vi "LJUD_ListAll.vi"(8 "error in":errorcluster, 9 "ConnectionType":i32=1, 10 "DeviceType":i32=9) -> (0 "error out":errorcluster, 1 "SerialNumbers":i32[](array[numeric]), 2 "NumFound":i32=2, 5 "Addresses":i32[](array[numeric]), 7 "IDs":i32[](array[numeric]))   [LabVIEW 2021]
doc: "Returns all the devices found of a given DeviceType and\nConnectionType. \n\nDocumented in Section 4.2 of the device's datasheet.\n\nDeviceType: LJ_dtU3=3, LJ_dtU6=6, LJ_dtUE9=9\n\nConnectionType: LJ_ctUSB=1, LJ_ctETHERNET=2"
uses:
  labjackud.dll
panel:
  # "Returns all the devices found of a given DeviceType and\nConnectionType. \n\nDocumented in Section 4.2 of the device's datasheet.\n\nDeviceType:  LJ_dtU3=3, LJ_dtU6=6, LJ_dtUE9=9\n\nConnectionType:  LJ_ctUSB=1, LJ_ctETHERNET=2"
  # "U3 = 3\nU6 = 6\nUE9 = 9\n \nUSB = 1\nETHERNET = 2"
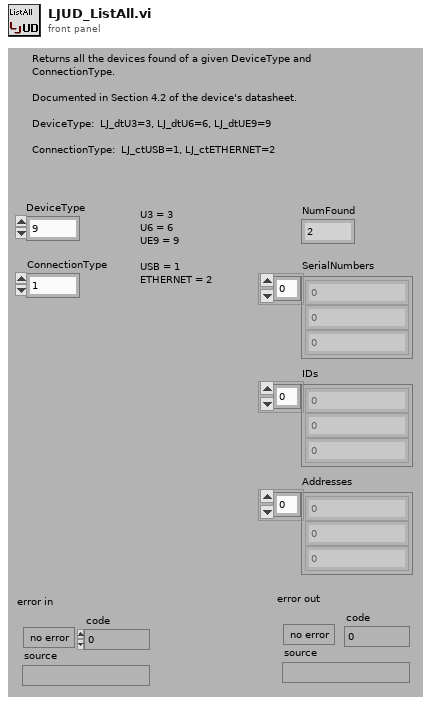
[diagram p1: front panel]
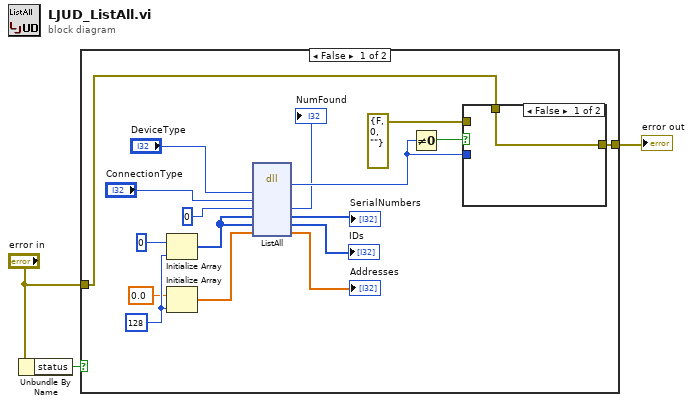
[diagram p0: block diagram]
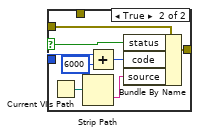
[diagram p2: hidden frame]
diagram:
  n1 = Unbundle By Name("error in") -> ("status"=w2:bool)
  n2 = case shown="False" w2 {
    tunnel: [w15 w30] -> w3
    tunnel: "error in" -> [w4 w30]
    frame False {
      w10 = 128 ("Dimension Size")
      n3 = Initialize Array(0 ("Element Data"), w10) -> (w7:i32[])
      n4 = Initialize Array(0.0 ("Element Data"), w10) -> (w6:dbl[])
      n5 = dll-call lib="labjackud.dll" fn="ListAll"("DeviceType"="DeviceType", "ConnectionType"="ConnectionType", "NumFound"=0, "SerialNumbers"=w7, "IDs"=w7, "Addresses"=w6) -> (w16:i32, "NumFound"=→"NumFound":i32, "SerialNumbers"=→"SerialNumbers":i32[], "IDs"=→"IDs":i32[], "Addresses"=→"Addresses":dbl[])  [unwired: 5 in, 2 out]
      n6 = Not Equal To 0?(x=w16) -> (x != 0?=w17:bool)
      n7 = case shown="False" w17 {
        selector: w17 -> [_ w28]
        tunnel: [w21 w29] -> w15
        tunnel: errorcluster {"status"=FALSE, "code"=0, "source"=""} ("error IO") -> [_ w27]
        tunnel: w16 -> [_ w23]
        tunnel: w4 -> [w21 _]
        frame False {
        }
        frame True {
          n8 = Current VI's Path() -> (path=w25:path)
          n9 = Strip Path(path=w25) -> (name=w26:string)  [unwired: 1 out]
          n10 = Add(x=w23, y=6000) -> (x+y=w24:i32)
          n11 = Bundle By Name(cluster=w27, "status"=w28, "code"=w24, "source"=w26) -> (w29:errorcluster)
        }
      }
    }
    frame True {
    }
  }
  "error out" <- w3
